vi "ReadCANStatus.vi"(8 "error in (no error)":errorcluster caption="错误输入（无错误）", 9 "CANInd":u32, 10 "DeciceInd":u32, 11 "DeviceType":u32) -> (0 "error out":errorcluster caption="错误输出", 2 "VCI_CAN_STATUS":T1, 3 "Valid":bool)   [LabVIEW 2011]
uses:
  data/ControlCAN.dll
panel:
  # "typedef struct _VCI_CAN_STATUS{\n\tUCHAR\tErrInterrupt;\n\tUCHAR\tregMode;\n\tUCHAR\tregStatus;\n\tUCHAR\tregALCapture;\n\tUCHAR\tregECCapture; \n\tUCHAR\tregEWLimit;\n\tUCHAR\tregRECounter; \n\tUCHAR\tregTECounter;\n\tDWORD\tReserved;\n}VCI_CAN_STATUS,*PVCI_CAN_STATUS;"
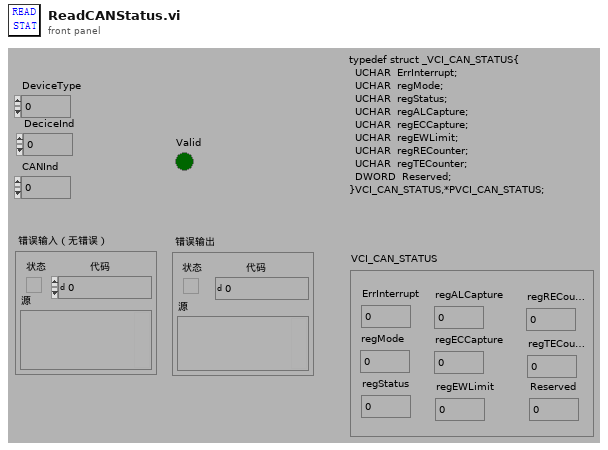
[diagram p1: front panel]
types:
  T1 = cluster{"ErrInterrupt":u8, "regMode":u8, "regStatus":u8, "regALCapture":u8, "regECCapture":u8, "regEWLimit":u8, "regRECounter":u8, "regTECounter":u8, "Reserved":u32}
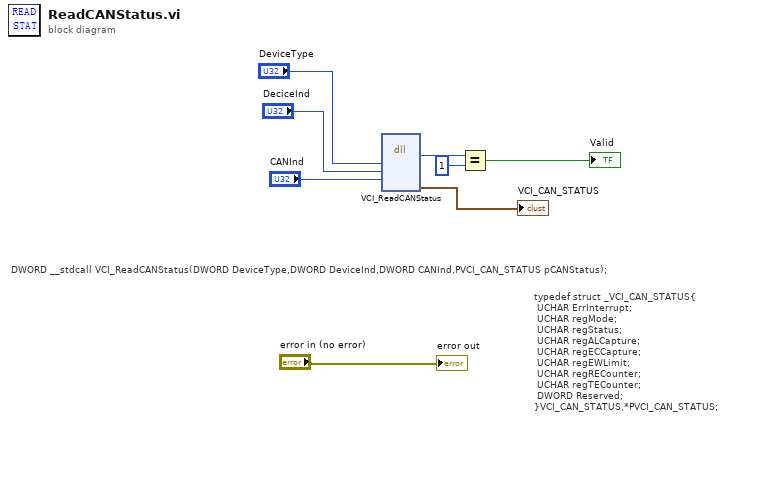
[diagram p0: block diagram]
diagram:
  # "typedef struct _VCI_CAN_STATUS{\n\tUCHAR\tErrInterrupt;\n\tUCHAR\tregMode;\n\tUCHAR\tregStatus;\n\tUCHAR\tregALCapture;\n\tUCHAR\tregECCapture; \n\tUCHAR\tregEWLimit;\n\tUCHAR\tregRECounter; \n\tUCHAR\tregTECounter;\n\tDWORD\tReserved;\n}VCI_CAN_STATUS,*PVCI_CAN_STATUS;"
  # "DWORD __stdcall VCI_ReadCANStatus(DWORD DeviceType,DWORD DeviceInd,DWORD CANInd,PVCI_CAN_STATUS pCANStatus);"
  n1 = dll-call lib="PTH1Nabs D\t董海成\t上位机2.进行中USB-CAN TooldataControlCAN.dll" fn="VCI_ReadCANStatus" label="VCI_StartCAN"("DeviceType"="DeviceType", "DeciceInd"="DeciceInd", "CANInd"="CANInd") -> ("返回类型"=w1:u32, "VCI_CAN_STATUS"=→"VCI_CAN_STATUS":T1)  [unwired: 7 in, 2 out]
  n2 = Equal?(x=w1, y=u32 1) -> (x = y?=→"Valid":bool)
  "error out" <- "error in (no error)"
